vi "Write to XML File(array).vi"(6 "Standalone? (T)":bool=TRUE, 8 "error in (no error)":errorcluster, 9 "XML Encoding":string, 10 "XML Input":string[](array[string]), 11 "XML File Path":path) -> (0 "error out":errorcluster, 2 "XML String":string, 3 "XML File Path":path)   [LabVIEW 2020]
doc: "Writes a text string of XML data with accompanying header tags to a text file. Wire data to the <B>XML Input</B> input to determine the polymorphic instance to use or manually select the instance. All XML data must follow the standard LabVIEW XML schema."
panel:
  in  "Prompt":string="Select Path to XML File"
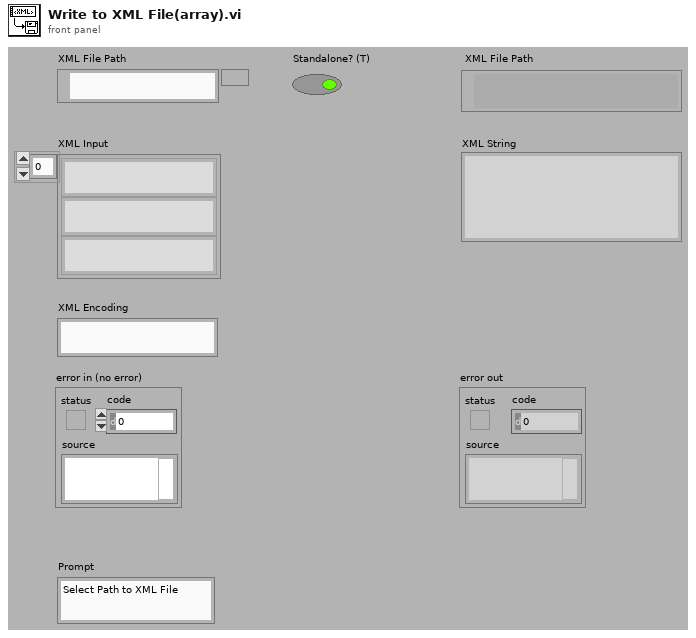
[diagram p1: front panel]
types:
  T1 = enum16{"open", "open or create", "create or replace", "create", "open (read only)"}
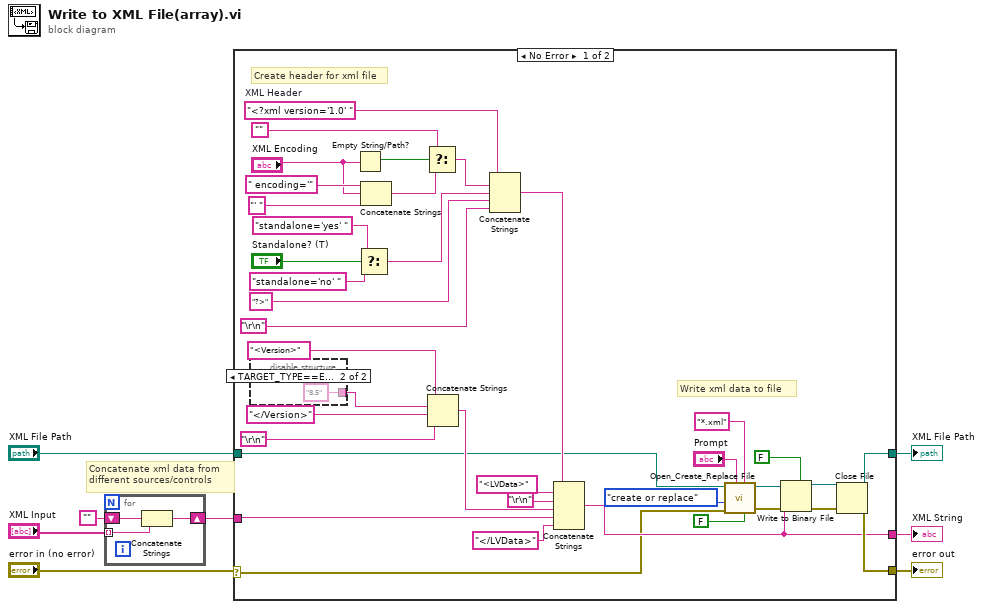
[diagram p0: block diagram]
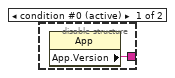
[diagram p2: hidden frame]
diagram:
  # "Concatenate xml data from\ndifferent sources/controls"
  n1 = for {
    tunnel: "XML Input" -> [w10] mode=indexing
    shift-right: [w9] -> w2
    shift-left: "" -> [w11]
    n2 = Concatenate Strings(w11, w10) -> (w9:string)
  }
  n3 = case shown="No Error" "error in (no error)" {
    selector: "error in (no error)" -> [w15 w54]
    tunnel: [w21 w54] -> w7
    tunnel: w2 -> [w18 w52]
    tunnel: [w19 w52] -> w6
    tunnel: "XML File Path" -> [w16 w53]
    tunnel: [w20 w53] -> w4
    frame No Error {
      w49 = "<?xml version='1.0' "  # XML Header
      # "Create header for xml file"
      # "Create header for xml file"
      # "Write xml data to file"
      n4 = disable-structure shown="TARGET_TYPE==Embedded||TARGET_TYPE==PocketPC" {
        disable-tunnel: [w50 "8.5" ("App.Version")] -> w32
        frame condition #0 (active) {
          n5 = property class="App"() -> ("App.Version"=w50:string)  [unwired: 2 in, 2 out]
        }
        frame condition #1 {
        }
      }
      n6 = Empty String/Path?(string/path="XML Encoding") -> (empty?=w40:bool)
      n7 = Select(t="standalone='yes' " ("Substring"), s="Standalone? (T)", f="standalone='no' " ("Substring")) -> (s? t:f=w34:string)
      n8 = Concatenate Strings(" encoding='", "XML Encoding", "' " ("Substring")) -> (w39:string)
      n9 = Select(t="", s=w40, f=w39) -> (s? t:f=w37:string)
      n10 = Concatenate Strings("<Version>", w32, "</Version>", "\r\n") -> (w29:string)
      n11 = Concatenate Strings(w49, w37, w34, "?>" ("Substring"), "\r\n") -> (w45:string)
      n12 = Concatenate Strings(w45, "<LVData>" ("Substring"), "\r\n", w29, w18, "</LVData>" ("Substring")) -> (w19:string)
      n13 = call "Open_Create_Replace File.vi"("advisory dialog? (display:T)"=FALSE, "pattern"="*.xml", "prompt"="Prompt", "error in (no error)"=w15, "function (open:0)"=T1."create or replace", "file path"=w16) -> ("error out"=w26:errorcluster, "refnum"=w14:refnum<file>)  [unwired: 2 in, 2 out]
      n14 = Write to Binary File(file (use dialog)=w14, data=w19, error in=w26, 5:FALSE ("prepend array or string size? (T)")) -> (refnum out=w23:refnum<file>, error out=w25:errorcluster)  [unwired: 3 out]
      n15 = Close File(refnum=w23, error in=w25) -> (path=w20:path, error out=w21:errorcluster)
    }
    frame Error {
    }
  }
  "error out" <- w7
  "XML String" <- w6
  "XML File Path" <- w4
